vi "L0_Initv2.vi"(8 "error in":errorcluster, 11 "connection ID in":refnum<k5>) -> (0 "error out":errorcluster, 3 "connection ID out":refnum<k5>)   [LabVIEW 2012]
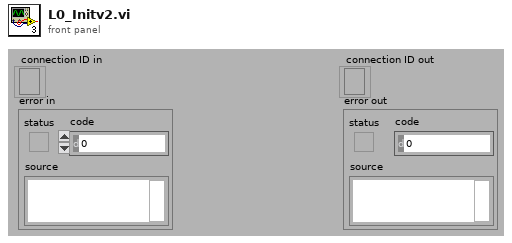
[diagram p1: front panel]
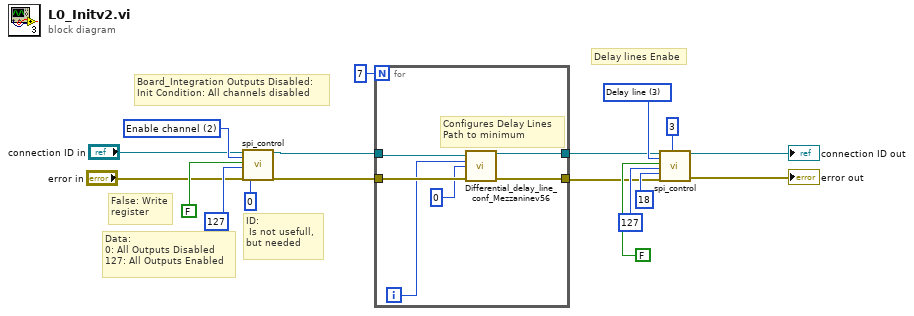
[diagram p0: block diagram]
diagram:
  w12 = u16 2 items=["Attenuation", "Clipping", "Enable channel", "Delay line", "ASIC"] ("Device")
  w15 = u16 3 items=["Attenuation", "Clipping", "Enable channel", "Delay line", "ASIC"] ("Device")
  # "False: Write\nregister"
  # "Data:\n0: All Outputs Disabled\n127: All Outputs Enabled"
  # "ID:\n Is not usefull, \nbut needed"
  # "Board_Integration Outputs Disabled:\nInit Condition: All channels disabled"
  # "Delay lines Enabe"
  n1 = call "spi_control.vi"("connection ID"="connection ID in", "Device"=w12, "Read/#write"=FALSE, "Data"=127, "error in"="error in", "Id in"=0) -> ("connection ID out"=w4:refnum<k5>, "error out 2"=w3:errorcluster)  [unwired: 6 in, 6 out]
  n2 = for {
    N: 7 -> [_]
    tunnel: w4 -> [w22]
    tunnel: [w23] -> w1
    tunnel: [w24] -> w2
    tunnel: w3 -> [w21]
    i -> [w20]
    # "Configures Delay Lines\nPath to minimum"
    n3 = call "Differential_delay_line_conf_Mezzaninev56.vi"("connection ID"=w22, "channel"=w20, "Delay value"=u16 0, "error in (no error)"=w21) -> ("connection ID out"=w23:refnum<k5>, "error out 2"=w24:errorcluster)  [unwired: 4 in, 6 out]
  }
  n4 = call "spi_control.vi"("connection ID"=w1, "Device"=w15, "Read/#write"=FALSE, "Data"=127, "Register or channel"=18, "error in"=w2, "chip delay"=3) -> ("connection ID out"=→"connection ID out":refnum<k5>, "error out 2"=→"error out":errorcluster)  [unwired: 5 in, 6 out]
